vi "Data Get Double.vi"(8 "error in (no error)":errorcluster, 11 "Data DVR in":refnum<data-value>) -> (0 "error out":errorcluster, 2 "DBL out":dbl, 3 "Data DVR out":refnum<data-value>)   [LabVIEW 2010, in "MDSplus.lvlib"]
doc: "Converts this data into a double. Implemented at this class level by returning TDI data(FT_FLOAT(this)). If data() fails or the returned class is not scalar, it generates an exception."
uses:
  <vilib>/MDSplus/Library/MDSplus.lvlib
  <vilib>/MDSplus/Classes/Data_Class/Data.lvclass
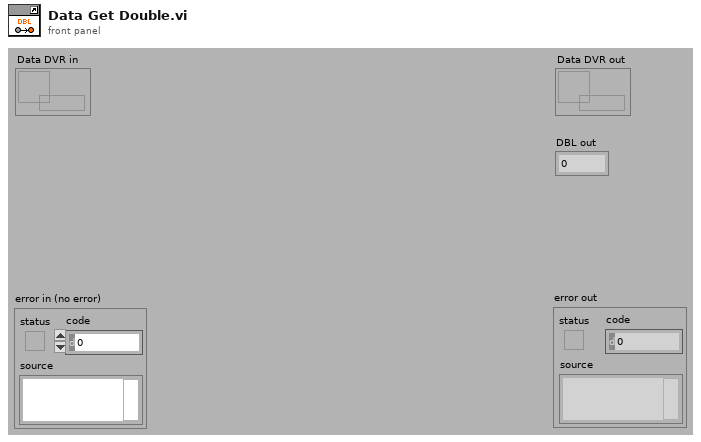
[diagram p1: front panel]
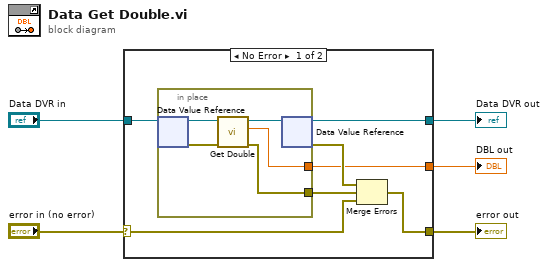
[diagram p0: block diagram]
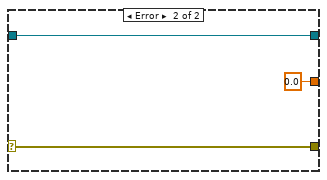
[diagram p2: hidden frame]
diagram:
  n1 = case shown="No Error" "error in (no error)" {
    selector: "error in (no error)" -> [w10 w19]
    tunnel: "Data DVR in" -> [w12 w18]
    tunnel: [w8 w19] -> w5
    tunnel: [w7 w18] -> w1
    tunnel: [w6 0.0 ("Float out")] -> w4
    frame No Error {
      n2 = in-place {
        in-place-border: [w15] -> w11
        in-place-border: [w13] -> w6
        n3 = in-place-dvr #1(w12) -> (w17:refnum<class "Data.lvclass">, w14:errorcluster)
        n4 = call-dynamic "Get Double.vi"("error in (no error)"=w14, "Data in"=w17) -> ("error out"=w15:errorcluster, "DBL out"=w13:dbl, "Data out"=w16:refnum<class "Data.lvclass">)  [unwired: 7 in]
        n5 = in-place-dvr #1(w16) -> (w7:refnum<data-value>, w9:errorcluster)
      }
      n6 = Merge Errors(w9, w11, w10) -> (w8:errorcluster)
    }
    frame Error {
    }
  }
  "error out" <- w5
  "DBL out" <- w4
  "Data DVR out" <- w1
